vi "potential_v2.vi"() -> ()   [LabVIEW 2009]
panel:
  out "Lennard-Jonson potential":cluster{"Y":dbl[], "Y":dbl[]}[](graph)
  in  "sig":ext(slide)=0.30659025787965616 scale=0.0..1.0
  in  "eps":ext(slide)=19.772727272727273 scale=30.0..0.0
  in  "stop":bool
  out "r":ext=1.000000000000000008
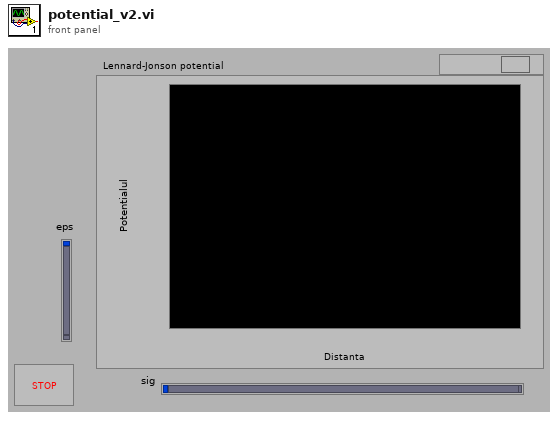
[diagram p1: front panel]
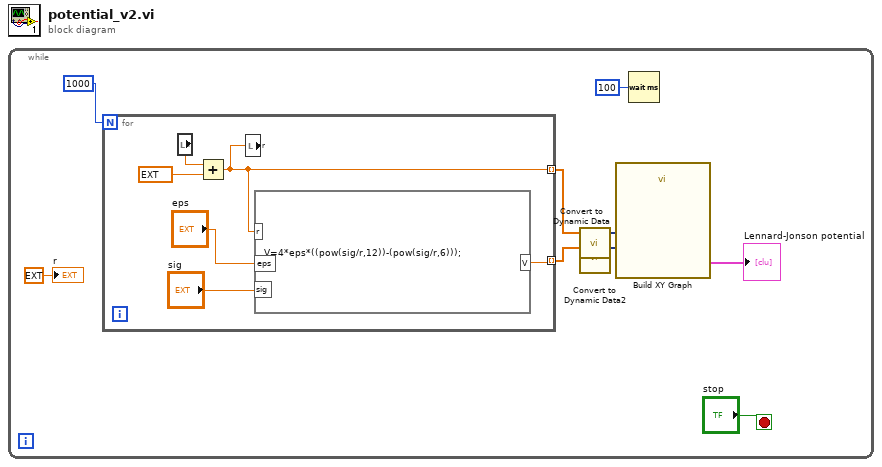
[diagram p0: block diagram]
diagram:
  n1 = while {
    stop <- "stop" stop-if-true
    n2 = for {
      N: 1000 -> [_]
      tunnel: [w10] -> w4 mode=indexing
      tunnel: [w14] -> w2 mode=indexing
      n3 = local read "r"() -> (w15:ext)
      n4 = Add(x=w15, y=ext 0.00099999999999999999996) -> (x+y=w10:ext)
      n5 = local write "r"(w10) -> ()
      n6 = formula code="V=4*eps*((pow(sig/r,12))-(pow(sig/r,6)));"("r"=w10, "eps"="eps", "sig"="sig") -> ("V"=w14:dbl)
    }
    n7 = call "Convert to Dynamic Data"("Array"=w4) -> ("Dynamic Data Type"=w3:dynamicdata)  [unwired: 3 in]
    n8 = call "Convert to Dynamic Data2"("Array"=w2) -> ("Dynamic Data Type"=w1:dynamicdata)  [unwired: 3 in]
    n9 = call "Build XY Graph"("Y Input"=w1, "X Input"=w3) -> ("XY Graph"=→"Lennard-Jonson potential":cluster{"Y":dbl[], "Y":dbl[]}[])  [unwired: 8 in, 1 out]
    n10 = Wait (ms)(milliseconds to wait=u32 100) -> ()  [unwired: 1 out]
    "r" <- ext 0.0 ("r")
  }
